vi "Handle Result.vi"(8 "error in (no error)":errorcluster, 10 "Result":T1={"Name"="", "Description"="", "Status"=enum."Passed", "Result Type"=enum."Test Suite", "Execution Time"=0.0, "Data"={"Expected"=variant, "Actual"=variant, "Delta"=variant}}, 11 "Text Report In":refnum<class "Text Report.lvclass">) -> (0 "error out":errorcluster, 3 "Text Report Out":refnum<class "Text Report.lvclass">)   [LabVIEW 2020, in "Reports.lvlib" / "Text Report.lvclass"]
uses:
  Text Report.lvclass
  Core/Result/Result.ctl
  Core/Result/Status.ctl
  Core/Result/Type.ctl
  Text Report.lvclass/Text Report.ctl
  Framework/Utilities/Utilities.lvlib
  Core/Result/Result.lvlib
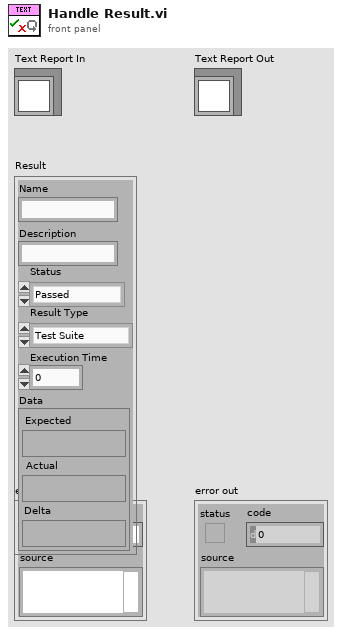
[diagram p1: front panel]
types:
  T1 = typedef "Result.lvlib/Result.ctl" = cluster{"Name":string, "Description":string, "Status":T2, "Result Type":T3, "Execution Time":dbl, "Data":cluster{"Expected":variant, "Actual":variant, "Delta":variant}}
  T2 = typedef "Result.lvlib/Status.ctl" = enum16{"", "Passed", "Failed", "Error", "Skipped", "Setup Error", "Broken", "Teardown Error"}
  T3 = typedef "Result.lvlib/Type.ctl" = enum16{"Test Case", "Test Suite", "Test Run", "Pass", "Fail", "Skip", "Pass if", "Fail if", "Pass if Error", "Fail if Error", "Pass if Equal", "Fail if Equal"}
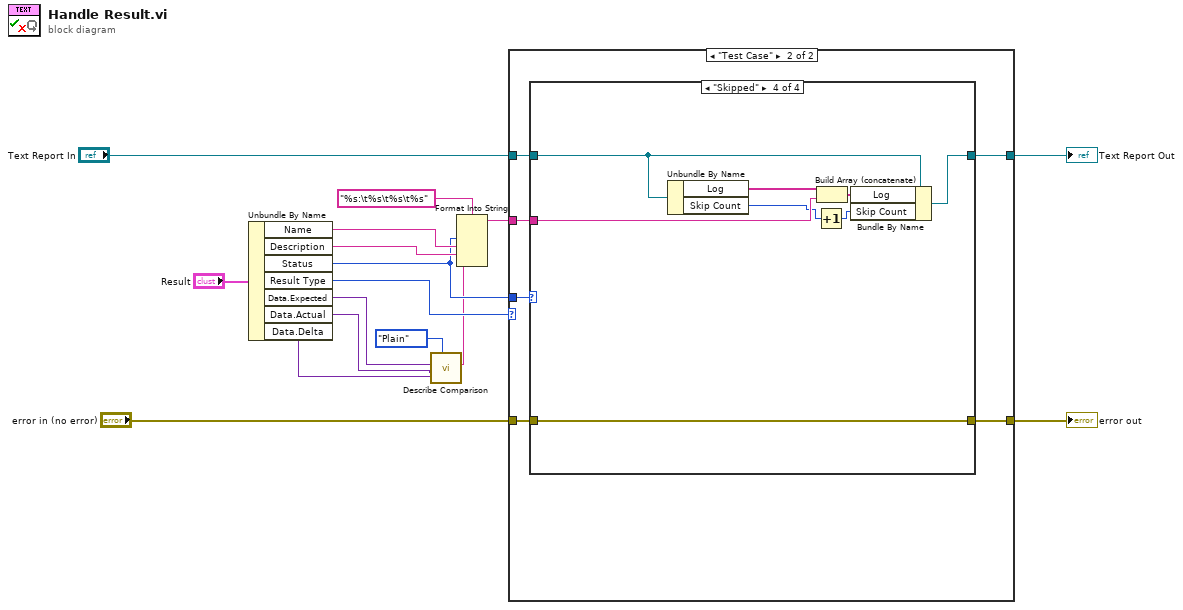
[diagram p0: block diagram]
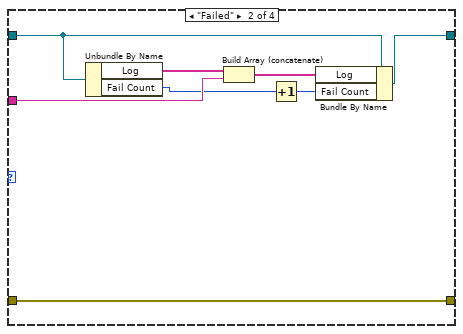
[diagram p4: hidden frame]
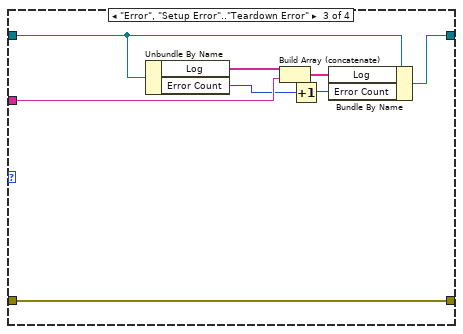
[diagram p5: hidden frame]
diagram:
  n1 = Unbundle By Name("Result") -> ("Name"=w12:string, "Description"=w11:string, "Status"=w9:T2, "Result Type"=w6:T3, "Data.Expected"=w5:variant, "Data.Actual"=w4:variant, "Data.Delta"=w3:variant)
  n2 = call "Describe Comparison.vi"("Delta"=w3, "Style"=enum16{"Diff", "Plain"}."Plain", "Actual"=w4, "Expected"=w5) -> ("Description"=w2:string)  [unwired: 7 in]
  n3 = Format Into String(format string="%s:\t%s\t%s\t%s", w9, w12, w11, w2) -> (resulting string=w10:string)  [unwired: 2 in, 1 out]
  n4 = case shown="\"Test Case\"" w6 {
    tunnel: "error in (no error)" -> [w17 w24]
    tunnel: [w17 w23] -> w15
    tunnel: w10 -> [_ w22]
    tunnel: w9 -> [_ w21]
    tunnel: "Text Report In" -> [w18 w20]
    tunnel: [w18 w19] -> w7
    frame Default {
    }
    frame "Test Case" {
      n5 = case shown="\"Skipped\"" w21 {
        tunnel: w24 -> [w26 w34 w42 w50]
        tunnel: [w26 w34 w42 w50] -> w23
        tunnel: w22 -> [_ w33 w41 w49]
        tunnel: w20 -> [w25 w31 w39 w47]
        tunnel: [w25 w29 w37 w45] -> w19
        frame "", Default {
        }
        frame "Failed" {
          n6 = Unbundle By Name(w31) -> ("Log"=w32:string[], "Fail Count"=w27:i32)
          n7 = Build Array (concatenate)(w32, w33) -> (w30:string[])
          n8 = Increment(x=w27) -> (x+1=w28:i32)
          n9 = Bundle By Name(cluster=w31, "Log"=w30, "Fail Count"=w28) -> (w29:refnum<class "Text Report.lvclass">)
        }
        frame "Error", "Setup Error".."Teardown Error" {
          n10 = Unbundle By Name(w39) -> ("Log"=w40:string[], "Error Count"=w35:i32)
          n11 = Build Array (concatenate)(w40, w41) -> (w38:string[])
          n12 = Increment(x=w35) -> (x+1=w36:i32)
          n13 = Bundle By Name(cluster=w39, "Log"=w38, "Error Count"=w36) -> (w37:refnum<class "Text Report.lvclass">)
        }
        frame "Skipped" {
          n14 = Unbundle By Name(w47) -> ("Log"=w48:string[], "Skip Count"=w43:i32)
          n15 = Increment(x=w43) -> (x+1=w44:i32)
          n16 = Build Array (concatenate)(w48, w49) -> (w46:string[])
          n17 = Bundle By Name(cluster=w47, "Log"=w46, "Skip Count"=w44) -> (w45:refnum<class "Text Report.lvclass">)
        }
      }
    }
  }
  "error out" <- w15
  "Text Report Out" <- w7
